vi "Punto 1 _ JUAN BERMUDEZ.vi"() -> ()   [LabVIEW 2020]
panel:
  out "Suma de pares de 100 a 2001":dbl
  out "Resta de pares e impares":dbl
  out "Suma de impares de 500 a 1500":dbl
  in  "Stop buttom":bool
  out "Suma de pares de 100 a 2000":dbl
  # "Programa 1"
  # "Realizar un programa que sume todos los números pares de 100 hasta 2000 y a este\nresultado restarlo con la suma de los números impares del 500 hasta el 1500, muestre\nen pantalla el resultado."
  # "Hecho por Juan Andrés Bermúdez Gómez"
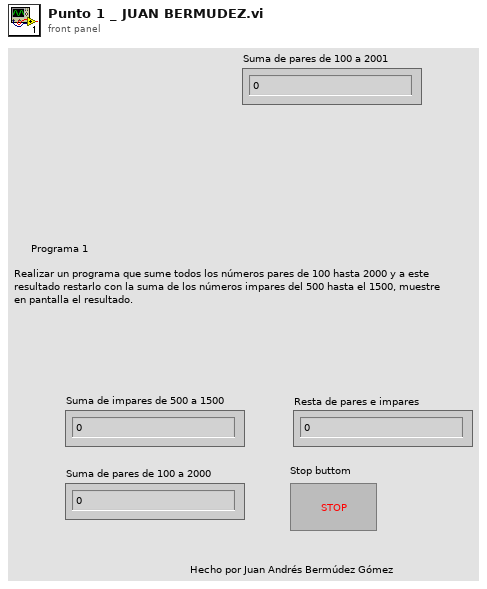
[diagram p1: front panel]
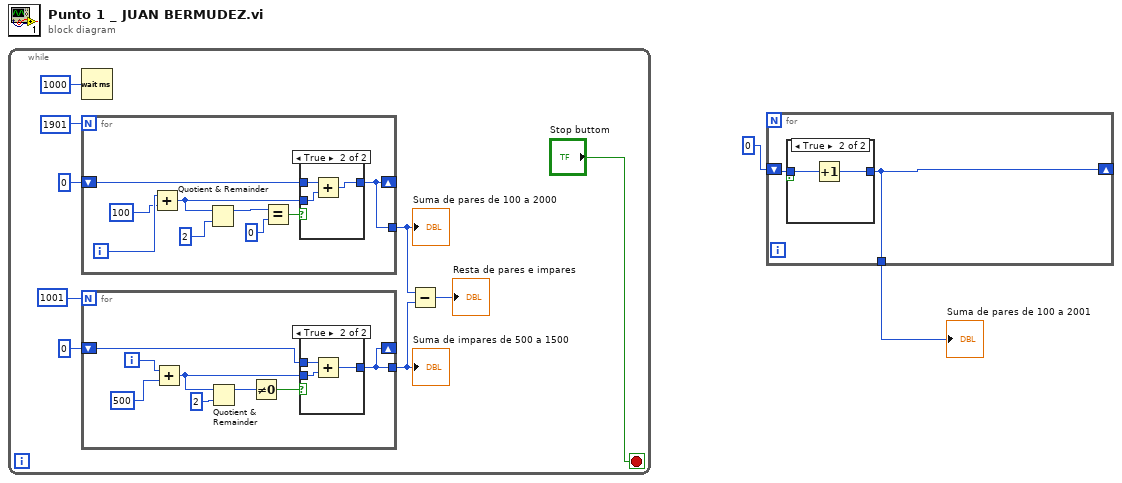
[diagram p0: block diagram]
diagram:
  n1 = while {
    stop <- "Stop buttom" stop-if-true
    n2 = Wait (ms)(milliseconds to wait=u32 1000) -> ()  [unwired: 1 out]
    n3 = for {
      N: 1901 -> [_]
      shift-right: [w24] -> _
      shift-left: 0 -> [w30]
      tunnel: [w24] -> w5
      i -> [w32]
      n4 = Add(x=w32, y=100) -> (x+y=w27:i32)
      n5 = Quotient & Remainder(x=w27, y=2) -> (x-y*floor(x/y)=w26:i32)  [unwired: 1 out]
      n6 = Equal?(x=w26, y=0) -> (x = y?=w25:bool)
      n7 = case shown="True" w25 {
        tunnel: w30 -> [w33 w36]
        tunnel: [w33 w35] -> w24
        tunnel: w27 -> [_ w34]
        frame False {
        }
        frame True {
          n8 = Add(x=w36, y=w34) -> (x+y=w35:i32)
        }
      }
    }
    "Suma de pares de 100 a 2000" <- w5
    n9 = for {
      N: 1001 -> [_]
      shift-right: [w12] -> _
      shift-left: 0 -> [w14]
      tunnel: [w12] -> w4
      i -> [w19]
      n10 = Add(x=w19, y=500) -> (x+y=w13:i32)
      n11 = Quotient & Remainder(x=w13, y=2) -> (x-y*floor(x/y)=w16:i32)  [unwired: 1 out]
      n12 = Not Equal To 0?(x=w16) -> (x != 0?=w15:bool)
      n13 = case shown="True" w15 {
        tunnel: w14 -> [w20 w23]
        tunnel: w13 -> [_ w22]
        tunnel: [w20 w21] -> w12
        frame False {
        }
        frame True {
          n14 = Add(x=w23, y=w22) -> (x+y=w21:i32)
        }
      }
    }
    "Suma de impares de 500 a 1500" <- w4
    n15 = Subtract(x=w5, y=w4) -> (x-y=→"Resta de pares e impares":i32)
  }
  n16 = for {
    shift-right: [w37] -> _
    shift-left: 0 -> [w38]
    tunnel: [w37] -> w1
    n17 = case shown="True" {
      selector: _ -> [_ _]
      tunnel: w38 -> [_ w40]
      tunnel: [_ w39] -> w37
      frame False {
      }
      frame True {
        n18 = Increment(x=w40) -> (x+1=w39:i32)
      }
    }
  }
  "Suma de pares de 100 a 2001" <- w1
